vi "RegWriteParams.vi"(5 "ScreenSetAvgg_Ref":refnum<vi>, 7 "InterlockExists_Ref":refnum<vi>, 8 "error IN":errorcluster, 9 "useShooter_Ref":refnum<vi>, 10 "useRecorder_Ref":refnum<vi>, 11 "useBallistician_Ref":refnum<vi>) -> (0 "errorOUT":errorcluster)   [LabVIEW 2010]
uses:
  <vilib>/registry/registry.llb/Registry RtKey.ctl
  <vilib>/registry/registry.llb/Registry SAM.ctl
  <vilib>/registry/registry.llb/Write Registry Value Simple STR.vi
panel:
  out "useShooter":string
  out "useRecorder":string
  out "useBallistician":string
  out "InterlockExist":string
  out "ScreenSetAveraging":string
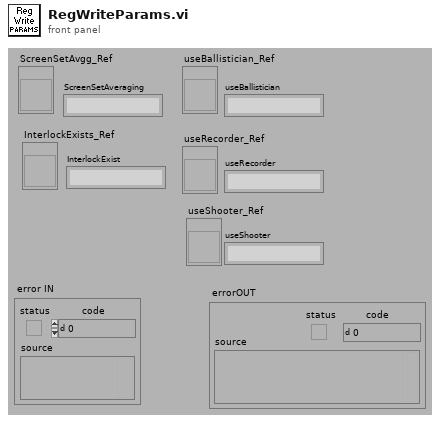
[diagram p1: front panel]
types:
  T1 = typedef "Registry RtKey.ctl" = enum32{"HKEY_CLASSES_ROOT", "HKEY_CURRENT_USER", "HKEY_LOCAL_MACHINE", "HKEY_USERS", "HKEY_PERFORMANCE_DATA", "HKEY_CURRENT_CONFIG", "HKEY_DYN_DATA"}
  T2 = typedef "Registry SAM.ctl" = enum32{"KEY_QUERY_VALUE", "KEY_SET_VALUE", "KEY_CREATE_SUB_KEY", "KEY_ENUMERATE_SUB_KEYS", "KEY_NOTIFY", "KEY_CREATE_LINK", "KEY_READ", "KEY_WRITE", "KEY_ALL_ACCESS", "KEY_READ | KEY_WRITE"}
  T3 = typedef "Registry refnum.ctl" = refnum<k1>
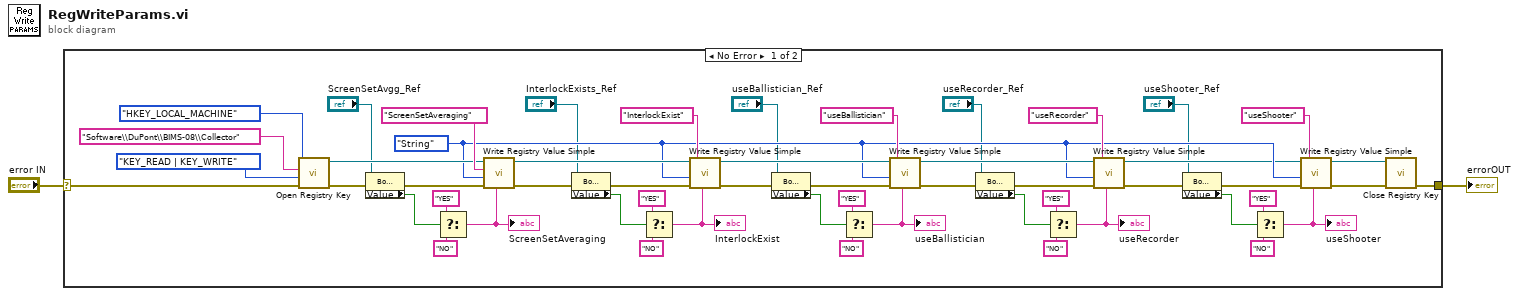
[diagram p0: block diagram]
diagram:
  n1 = case shown="No Error" "error IN" {
    selector: "error IN" -> [w52 w56]
    tunnel: [w51 w56] -> w1
    frame No Error {
      w12 = enum16{"String", "Binary", "DWORD"}."String" ("simple data type")
      n2 = call <vilib>:"Open Registry Key.vi"("error in (no error)"=w52, "security access mask (KEY_READ | KEY_WRITE)"=Registry_SAM."KEY_READ | KEY_WRITE", "subkey"="Software\\DuPont\\BIMS-08\\Collector", "root key (HKEY_LOCAL_MACHINE)"=Registry_RtKey."HKEY_LOCAL_MACHINE") -> ("error out"=w44:errorcluster, "refnum out"=w43:T3)  [unwired: 6 out]
      n3 = property on="Property Node" class="Bool (strict)"(reference="ScreenSetAvgg_Ref", error in=w44) -> (error out=w49:errorcluster, "Value"=w48:bool)  [unwired: 1 out]
      n4 = Select(t="YES", s=w48, f="NO") -> (s? t:f=w45:string)
      "ScreenSetAveraging" <- w45
      n5 = call-poly <vilib>:"Write Registry Value Simple.vi"("String/Binary data"=w45, "error in (no error)"=w49, "simple data type"=w12, "value"="ScreenSetAveraging", "refnum"=w43) -> ("error out"=w36:errorcluster, "refnum out"=w35:T3)  [unwired: 3 out]
      n6 = property on="Property Node" class="Bool (strict)"(reference="InterlockExists_Ref", error in=w36) -> (error out=w38:errorcluster, "Value"=w39:bool)  [unwired: 1 out]
      n7 = Select(t="YES", s=w39, f="NO") -> (s? t:f=w42:string)
      "InterlockExist" <- w42
      n8 = call-poly <vilib>:"Write Registry Value Simple.vi"("String/Binary data"=w42, "error in (no error)"=w38, "simple data type"=w12, "value"="InterlockExist", "refnum"=w35) -> ("error out"=w20:errorcluster, "refnum out"=w22:T3)  [unwired: 3 out]
      n9 = property on="Property Node" class="Bool (strict)"(reference="useBallistician_Ref", error in=w20) -> (error out=w33:errorcluster, "Value"=w32:bool)  [unwired: 1 out]
      n10 = Select(t="YES", s=w32, f="NO") -> (s? t:f=w29:string)
      "useBallistician" <- w29
      n11 = call-poly <vilib>:"Write Registry Value Simple.vi"("String/Binary data"=w29, "error in (no error)"=w33, "simple data type"=w12, "value"="useBallistician", "refnum"=w22) -> ("error out"=w19:errorcluster, "refnum out"=w21:T3)  [unwired: 3 out]
      n12 = property on="Property Node" class="Bool (strict)"(reference="useRecorder_Ref", error in=w19) -> (error out=w24:errorcluster, "Value"=w25:bool)  [unwired: 1 out]
      n13 = Select(t="YES", s=w25, f="NO") -> (s? t:f=w28:string)
      "useRecorder" <- w28
      n14 = call-poly <vilib>:"Write Registry Value Simple.vi"("String/Binary data"=w28, "error in (no error)"=w24, "simple data type"=w12, "value"="useRecorder", "refnum"=w21) -> ("error out"=w9:errorcluster, "refnum out"=w11:T3)  [unwired: 3 out]
      n15 = property on="Property Node" class="Bool (strict)"(reference="useShooter_Ref", error in=w9) -> (error out=w17:errorcluster, "Value"=w16:bool)  [unwired: 1 out]
      n16 = Select(t="YES", s=w16, f="NO") -> (s? t:f=w13:string)
      "useShooter" <- w13
      n17 = call-poly <vilib>:"Write Registry Value Simple.vi"("String/Binary data"=w13, "error in (no error)"=w17, "simple data type"=w12, "value"="useShooter", "refnum"=w11) -> ("error out"=w8:errorcluster, "refnum out"=w10:T3)  [unwired: 3 out]
      n18 = call <vilib>:"Close Registry Key.vi"("error in (no error)"=w8, "refnum"=w10) -> ("error out"=w51:errorcluster)  [unwired: 5 out]
    }
    frame Error {
    }
  }
  "errorOUT" <- w1
